vi "Shooter and Reload.vi"(0 "Shooter at bottom limit":T5, 5 "Winch Shifter Servo":T1={"DeviceStatus"={"status"=FALSE, "code"=0, "source"=""}, "Digital Module"=enum."Digital Module 1", "PWM Channel"=enum."Invalid", "DeadBand"={"Name"="", "maxPositivePwm"=0, "minPositivePwm"=0, "centerPwm"=0, "maxNegativePwm"=0, "minNegativePwm"=0, "angularRange"=0}}, 7 "LatchControlDevRef":T8={"DeviceStatus"={"status"=FALSE, "code"=0, "source"=""}, "Type"=enum."PWM", "PWM"={"Digital Module"=enum."Digital Module 1", "PWM Channel"=enum."Invalid", "DeadBand"={"Name"="", "maxPositivePwm"=0, "minPositivePwm"=0, "centerPwm"=0, "maxNegativePwm"=0, "minNegativePwm"=0, "angularRange"=0}}, "CAN"={"Device Number"=0, "Control Mode"=enum."Percent VBus", "Semaphore"=refnum, "Max Vout"=12.0}, "Invert"=FALSE, "TransformRef"=refnum, "InvTransformRef"=refnum}, 9 "ServoDeviceRef":T1={"DeviceStatus"={"status"=FALSE, "code"=0, "source"=""}, "Digital Module"=enum."Digital Module 1", "PWM Channel"=enum."Invalid", "DeadBand"={"Name"="", "maxPositivePwm"=0, "minPositivePwm"=0, "centerPwm"=0, "maxNegativePwm"=0, "minNegativePwm"=0, "angularRange"=0}}, 11 "ShooterWinchRef":T8={"DeviceStatus"={"status"=FALSE, "code"=0, "source"=""}, "Type"=enum."PWM", "PWM"={"Digital Module"=enum."Digital Module 1", "PWM Channel"=enum."Invalid", "DeadBand"={"Name"="", "maxPositivePwm"=0, "minPositivePwm"=0, "centerPwm"=0, "maxNegativePwm"=0, "minNegativePwm"=0, "angularRange"=0}}, "CAN"={"Device Number"=0, "Control Mode"=enum."Percent VBus", "Semaphore"=refnum, "Max Vout"=12.0}, "Invert"=FALSE, "TransformRef"=refnum, "InvTransformRef"=refnum}, 12 "Shooter Latch Sensors":T7) -> ()   [LabVIEW 2014]
uses:
  <vilib>/Rock Robotics/WPI/DigitalInput/WPI_DigitalInputDevRef.ctl
  <vilib>/Rock Robotics/SystemInterfaces/DIO/FPGA_DIOChannel.ctl
  <vilib>/Rock Robotics/SystemInterfaces/Typedef/FPGA_TypedefDigitalModule.ctl
  <vilib>/Rock Robotics/WPI/MotorControl/WPI_MotorControlDeviceRef.ctl
  <vilib>/Rock Robotics/SystemInterfaces/DIO/FPGA_DIOPWMChannel.ctl
  <vilib>/Rock Robotics/WPI/PWM/WPI_PWMDeadband.ctl
  <vilib>/Rock Robotics/WPI/CAN/Jaguar/SubVIs/WPI_CANJaguar_ControlMode.ctl
  <vilib>/Rock Robotics/WPI/PWM/WPI_PWMTransform_ConPane.ctl
  <vilib>/Rock Robotics/WPI/PWM/Servo/WPI_ServoDeviceRef.ctl
  Shoot and reload typedef.ctl
  Events.vi
panel:
  out "Shooter Latch Sensor Bottom":bool
  out "Shooter Latch Sensor Top":bool
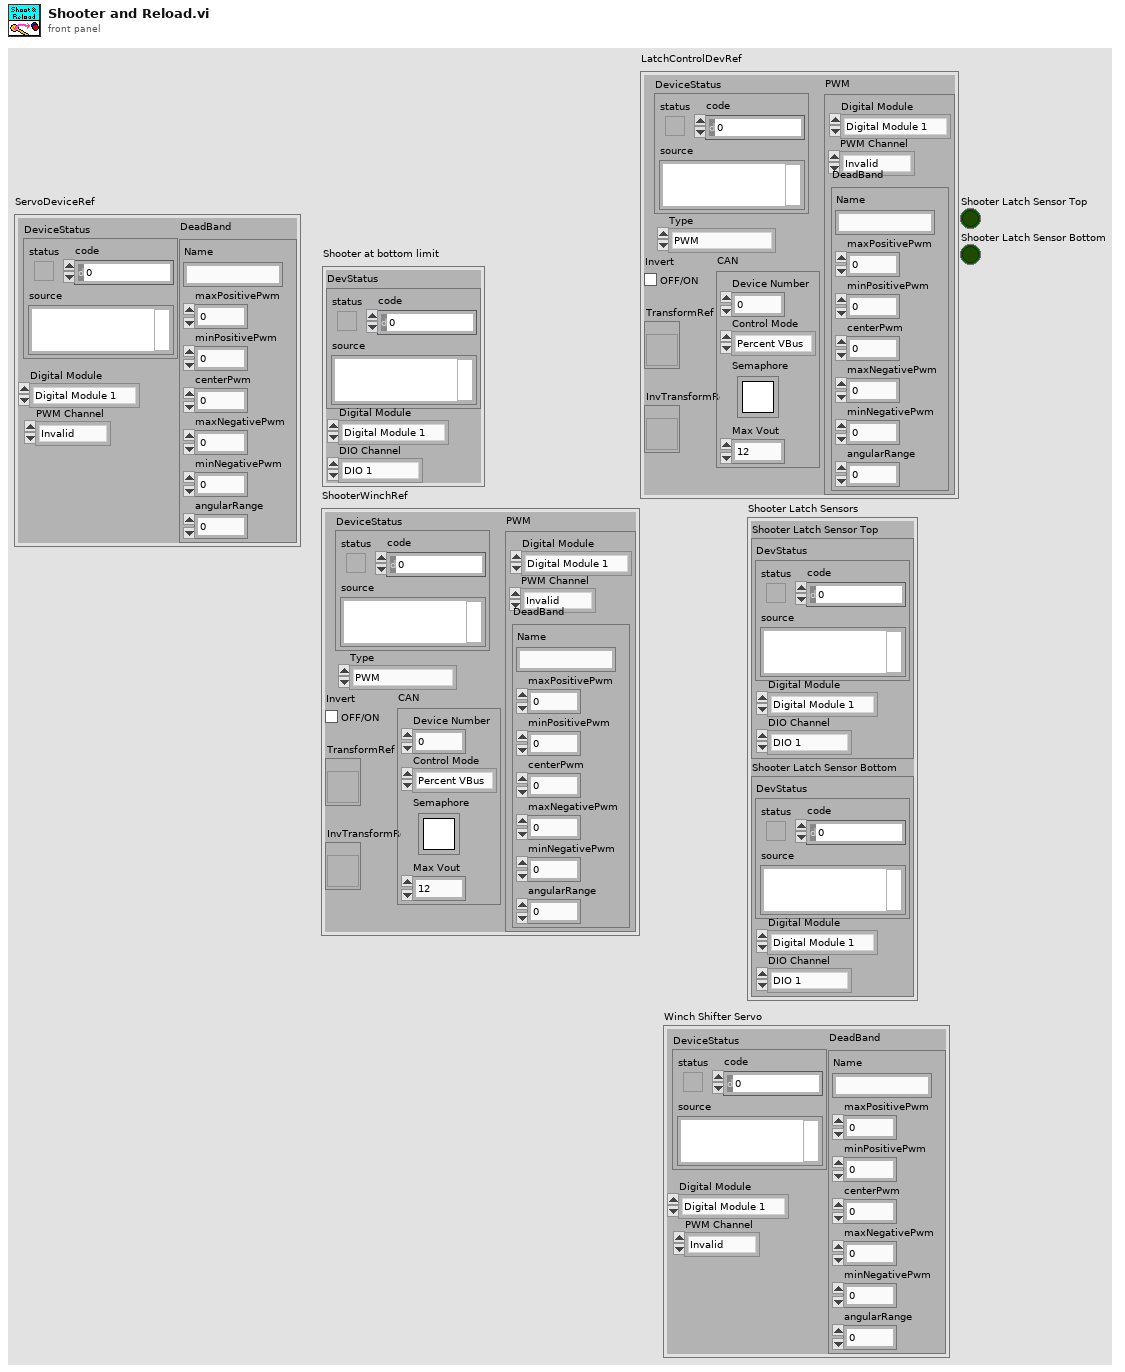
[diagram p1: front panel]
types:
  T1 = typedef "WPI_ServoDeviceRef.ctl" = cluster{"DeviceStatus":errorcluster, "Digital Module":T2, "PWM Channel":T3, "DeadBand":T4}
  T2 = typedef "FPGA_TypedefDigitalModule.ctl" = enum16{"Digital Module 1", "Digital Module 2"}
  T3 = typedef "FPGA_DIOPWMChannel.ctl" = enum8{"PWM 1", "PWM 2", "PWM 3", "PWM 4", "PWM 5", "PWM 6", "PWM 7", "PWM 8", "PWM 9", "PWM 10", "Invalid"}
  T4 = typedef "WPI_PWMDeadband.ctl" = cluster{"Name":string, "maxPositivePwm":i32, "minPositivePwm":i32, "centerPwm":i32, "maxNegativePwm":i32, "minNegativePwm":i32, "angularRange":u16}
  T5 = typedef "WPI_DigitalInputDevRef.ctl" = cluster{"DevStatus":errorcluster, "DIO Channel":T6, "Digital Module":T2}
  T6 = typedef "FPGA_DIOChannel.ctl" = enum8{"DIO 1", "DIO 2", "DIO 3", "DIO 4", "DIO 5", "DIO 6", "DIO 7", "DIO 8", "DIO 9", "DIO 10", "DIO 11", "DIO 12", "DIO 13", "DIO 14", "Invalid"}
  T7 = cluster{"Shooter Latch Sensor Top":T5, "Shooter Latch Sensor Bottom":T5}
  T8 = typedef "WPI_MotorControlDeviceRef.ctl" = cluster{"DeviceStatus":errorcluster, "Type":enum16{"PWM", "CAN"}, "PWM":cluster{"Digital Module":T2, "PWM Channel":T3, "DeadBand":T4}, "CAN":cluster{"Device Number":u8, "Control Mode":T9, "Semaphore":T10, "Max Vout":dbl}, "Invert":bool, "TransformRef":T11, "InvTransformRef":T11}
  T9 = typedef "WPI_CANJaguar_ControlMode.ctl" = enum8{"Percent VBus", "Current", "Speed", "Position", "Voltage"}
  T10 = typedef "Semaphore RefNum" = refnum<k1>
  T11 = typedef "WPI_PWMTransform_ConPane.ctl" = refnum<vi>
  T12 = typedef "Shoot and reload typedef.ctl" = enum16{"Wait for fire button", "First call", "Release Latch", "Wait for reload to be needed", "Engage gearbox", "Run motor", "Engage latch / Stall motor", "Stop motor", "truss shot servos", "Disengage Gearbox"}
  T13 = cluster{"axis 1":dbl, "axis 2":dbl, "axis 3":dbl, "axis 4":dbl, "axis 5":dbl, "Change Power":dbl}
  T14 = cluster{"Reloading?":bool, "Throw":bool, "Ready?":bool, "Truss throw":bool, "Power is high?":bool, "Automatic relaod?":bool, "Manuall servo":bool}
  T15 = typedef "Eventgrab.ctl" = cluster{"Grab":bool, "GroundPass":bool, "Test Aqaure":dbl, "Shoulder up or down?":bool, "Auton drag":bool}
  T16 = cluster{"Shooter latch power":dbl, "Shooter winch power":dbl, "Shooter gearbox servo angles disengaged":i32, "Shooter gearbox servo angles engaged":i32, "Shooter winch power while stalling":dbl, "Exponential Drive Exponent":dbl}
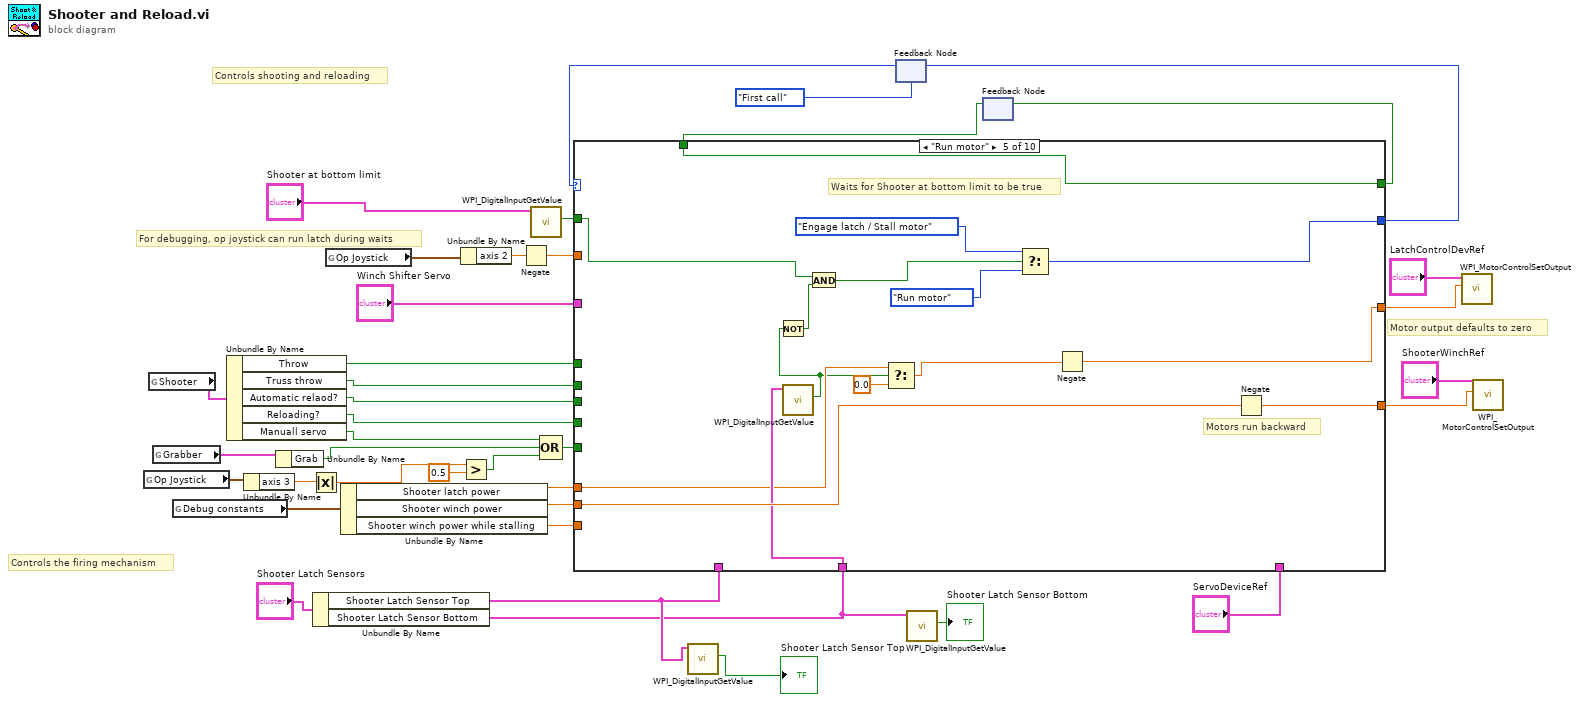
[diagram p0: block diagram]
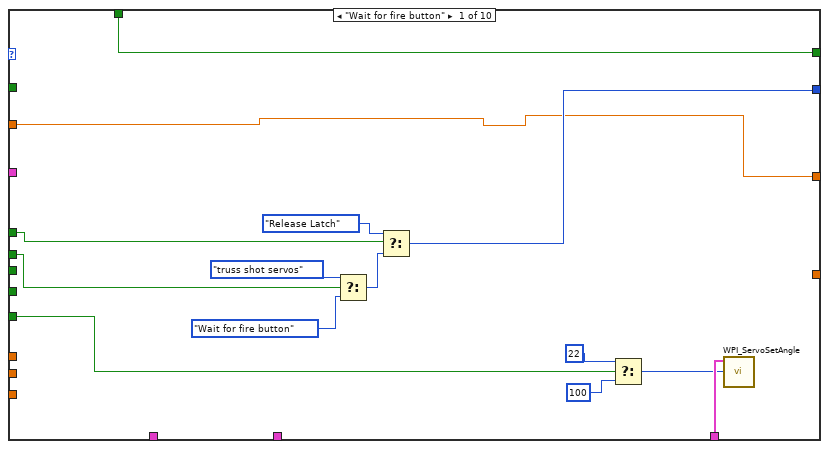
[diagram p2: hidden frame]
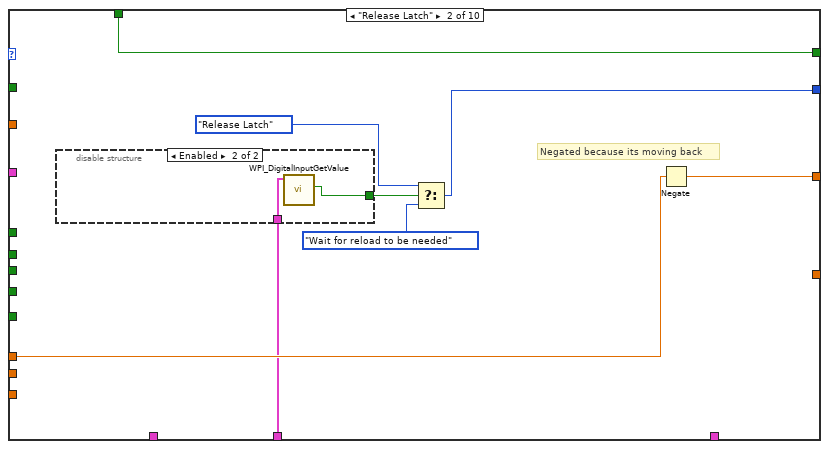
[diagram p3: hidden frame]
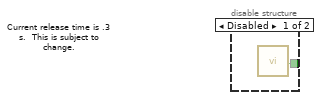
[diagram p4: hidden frame]
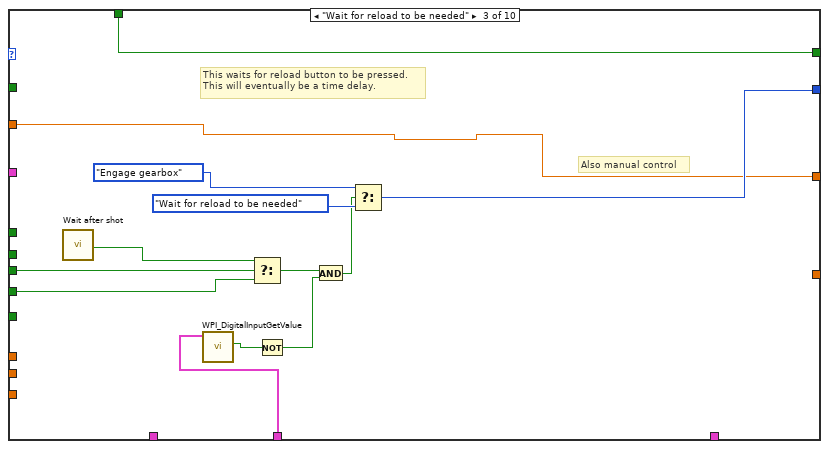
[diagram p5: hidden frame]
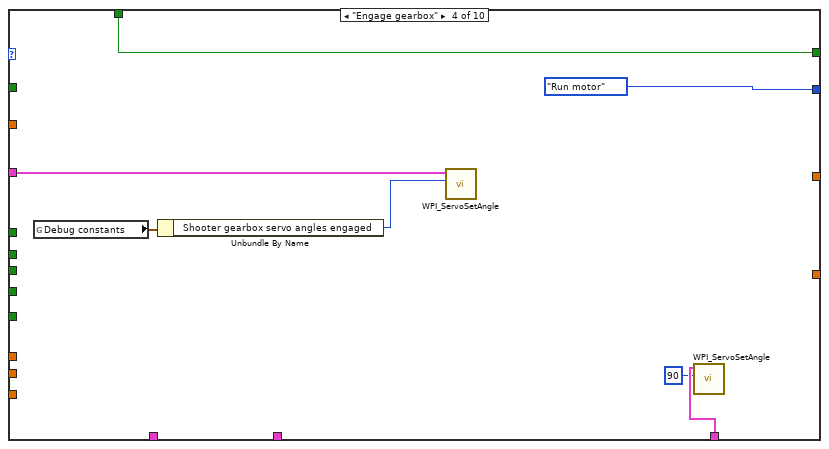
[diagram p6: hidden frame]
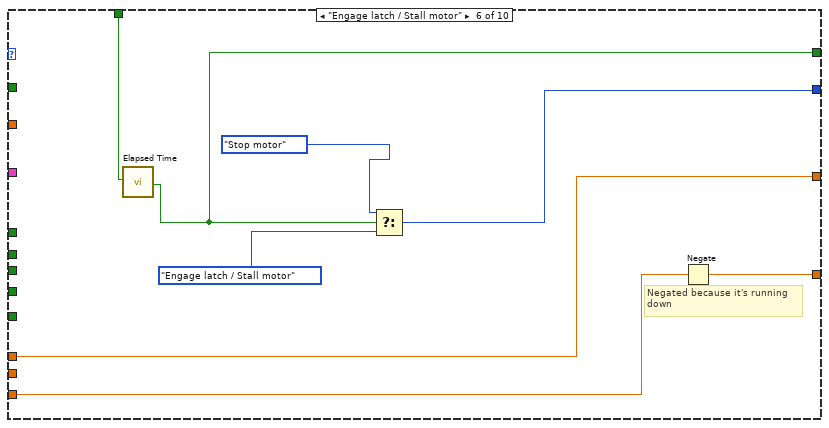
[diagram p7: hidden frame]
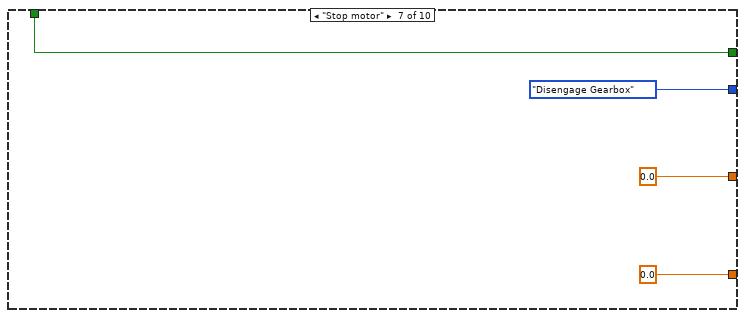
[diagram p8: hidden frame]
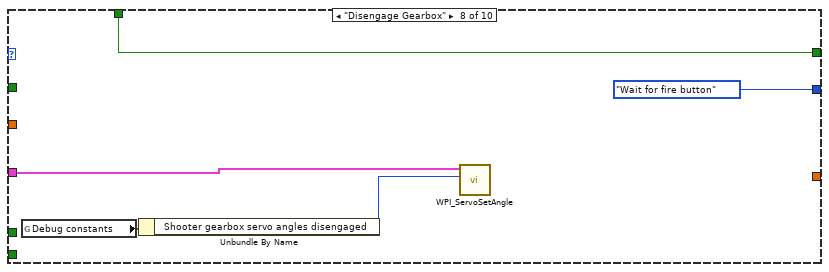
[diagram p9: hidden frame]
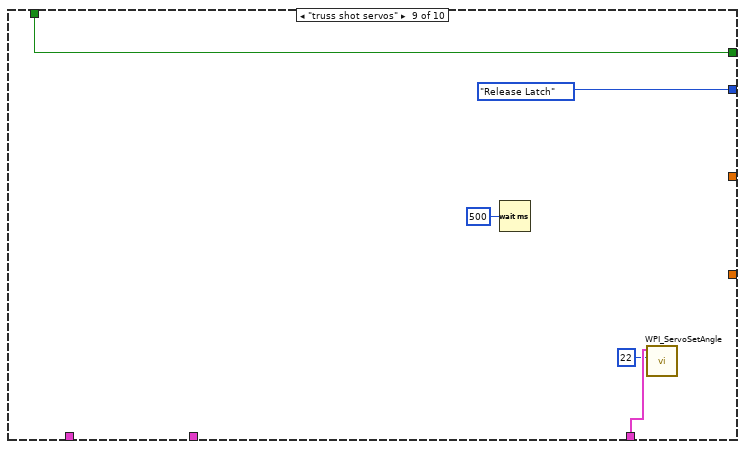
[diagram p10: hidden frame]
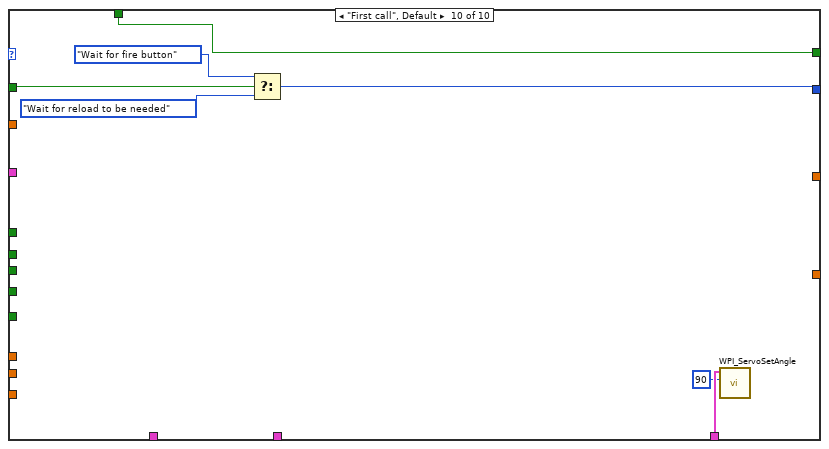
[diagram p11: hidden frame]
diagram:
  # "For debugging, op joystick can run latch during waits"
  # "Motor output defaults to zero"
  # "Controls the firing mechanism"
  # "Controls shooting and reloading"
  n1 = global read "Events.vi" "Op Joystick"() -> (w10:T13)
  n2 = global read "Events.vi" "Shooter"() -> (w39:T14)
  n3 = global read "Events.vi" "Grabber"() -> (w11:T15)
  n4 = global read "Events.vi" "Debug constants"() -> (w24:T16)
  n5 = Unbundle By Name(w39) -> ("Throw"=w14:bool, "Truss throw"=w13:bool, "Automatic relaod?"=w17:bool, "Reloading?"=w25:bool, "Manuall servo"=w6:bool)
  n6 = Unbundle By Name(w10) -> ("axis 3"=w9:dbl)
  n7 = Unbundle By Name(w11) -> ("Grab"=w5:bool)
  n8 = Absolute Value(x=w9) -> (abs(x)=w8:dbl)
  n9 = Unbundle By Name("Shooter Latch Sensors") -> ("Shooter Latch Sensor Top"=w18:T5, "Shooter Latch Sensor Bottom"=w16:T5)
  n10 = global read "Events.vi" "Op Joystick"() -> (w28:T13)
  n11 = Unbundle By Name(w24) -> ("Shooter latch power"=w23:dbl, "Shooter winch power"=w22:dbl, "Shooter winch power while stalling"=w21:dbl)
  n12 = Unbundle By Name ("ubn")(w28) -> ("axis 2"=w27:dbl)
  n13 = Greater?(x=w8, y=0.5) -> (0:w4:bool)
  n14 = Negate(x=w27) -> (-x=w26:dbl)
  n15 = call <vilib>:"WPI_DigitalInputGetValue.vi"("DigitalInputDevRef"="Shooter at bottom limit") -> ("Value"=w36:bool)  [unwired: 8 in, 2 out]
  n16 = Compound Arithmetic op=OR(w6, w5, w4) -> (w3:bool)
  n17 = call <vilib>:"WPI_DigitalInputGetValue.vi"("DigitalInputDevRef"=w18) -> ("Value"=→"Shooter Latch Sensor Top":bool)  [unwired: 8 in, 2 out]
  n18 = feedback #1(Shoot_and_reload_typedef."First call") -> (w34:T12)
  n19 = call <vilib>:"WPI_DigitalInputGetValue.vi"("DigitalInputDevRef"=w16) -> ("Value"=→"Shooter Latch Sensor Bottom":bool)  [unwired: 8 in, 2 out]
  n20 = feedback #2() -> (w2:bool)  [unwired: 1 in]
  n21 = case shown="\"Run motor\"" w34 {
    tunnel: w36 -> [_ _ _ _ w93 _ _ _ _ w128]
    tunnel: [w53 w60 w77 Shoot_and_reload_typedef."Run motor" w99 w107 Shoot_and_reload_typedef."Disengage Gearbox" ("f") Shoot_and_reload_typedef."Wait for fire button" ("f") Shoot_and_reload_typedef."Release Latch" ("f") w127] -> w35
    tunnel: [w41 w55 w66 _ w86 w104 0.0 _ _ _] -> w32
    tunnel: w25 -> [_ _ w74 _ _ _ _ _ _ _]
    tunnel: "Winch Shifter Servo" -> [_ _ _ w84 _ _ _ w116 _ _]
    tunnel: [_ _ _ _ w95 w106 0.0 ("Output") _ _ _] -> w29
    tunnel: w26 -> [w41 _ w66 _ _ _ _ _ _ _]
    tunnel: w23 -> [_ w57 _ _ w91 w104 _ _ _ _]
    tunnel: w22 -> [_ _ _ _ w96 _ _ _ _ _]
    tunnel: w21 -> [_ _ _ _ _ w105 _ _ _ _]
    tunnel: w18 -> [_ _ _ _ _ _ _ _ _ _]
    tunnel: w16 -> [_ w56 w67 _ w94 _ _ _ _ _]
    tunnel: w17 -> [_ _ w73 _ _ _ _ _ _ _]
    tunnel: w14 -> [w51 _ _ _ _ _ _ _ _ _]
    tunnel: w13 -> [w47 _ _ _ _ _ _ _ _ _]
    tunnel: "ServoDeviceRef" -> [w46 _ _ w80 _ _ _ _ w121 w124]
    tunnel: w3 -> [w42 _ _ _ _ _ _ _ _ _]
    tunnel: [w40 w54 w65 w78 w85 w101 w108 w112 w117 w122] -> w1
    tunnel: w2 -> [w40 w54 w65 w78 w85 w100 w108 w112 w117 w122]
    frame "Wait for fire button" {
      n22 = Select(t=Shoot_and_reload_typedef."truss shot servos", s=w47, f=Shoot_and_reload_typedef."Wait for fire button") -> (s? t:f=w49:T12)
      n23 = Select(t=Shoot_and_reload_typedef."Release Latch", s=w51, f=w49) -> (s? t:f=w53:T12)
      n24 = Select(t=22, s=w42, f=100) -> (s? t:f=w44:i32)
      n25 = call <vilib>:"WPI_ServoSetAngle.vi"("Angle"=w44, "ServoDeviceRef"=w46) -> ()  [unwired: 8 in, 2 out]
    }
    frame "Release Latch" {
      # "Negated because its moving back"
      n26 = disable-structure shown="Enabled" {
        disable-tunnel: [w62 w64] -> w61
        disable-tunnel: w56 -> [_ w63]
        frame Disabled {
          n27 = call "Current release time is .3 s.  This is subject to change."() -> ("Time has Elapsed"=w62:bool)  [unwired: 12 in, 7 out]
        }
        frame Enabled {
          n28 = call <vilib>:"WPI_DigitalInputGetValue.vi"("DigitalInputDevRef"=w63) -> ("Value"=w64:bool)  [unwired: 8 in, 2 out]
        }
      }
      n29 = Select(t=Shoot_and_reload_typedef."Release Latch", s=w61, f=Shoot_and_reload_typedef."Wait for reload to be needed") -> (s? t:f=w60:T12)
      n30 = Negate(x=w57) -> (-x=w55:dbl)
    }
    frame "Wait for reload to be needed" {
      # "Also manual control"
      # "This waits for reload button to be pressed.\nThis will eventually be a time delay."
      n31 = call "Wait after shot"() -> ("Time has Elapsed"=w72:bool)  [unwired: 12 in, 7 out]
      n32 = call <vilib>:"WPI_DigitalInputGetValue.vi"("DigitalInputDevRef"=w67) -> ("Value"=w68:bool)  [unwired: 8 in, 2 out]
      n33 = Select(t=w72, s=w73, f=w74) -> (s? t:f=w70:bool)
      n34 = Not(x=w68) -> (.not. x?=w71:bool)
      n35 = And(x=w70, y=w71) -> (x .and. y?=w69:bool)
      n36 = Select(t=Shoot_and_reload_typedef."Engage gearbox", s=w69, f=Shoot_and_reload_typedef."Wait for reload to be needed") -> (s? t:f=w77:T12)
    }
    frame "Engage gearbox" {
      n37 = global read "Events.vi" "Debug constants"() -> (w82:T16)
      n38 = Unbundle By Name(w82) -> ("Shooter gearbox servo angles engaged"=w81:i32)
      n39 = call <vilib>:"WPI_ServoSetAngle.vi"("Angle"=w81, "ServoDeviceRef"=w84) -> ()  [unwired: 8 in, 2 out]
      n40 = call <vilib>:"WPI_ServoSetAngle.vi"("Angle"=90, "ServoDeviceRef"=w80) -> ()  [unwired: 8 in, 2 out]
    }
    frame "Run motor" {
      # "Motors run backward"
      # "Waits for Shooter at bottom limit to be true"
      n41 = call <vilib>:"WPI_DigitalInputGetValue.vi"("DigitalInputDevRef"=w94) -> ("Value"=w89:bool)  [unwired: 8 in, 2 out]
      n42 = Not(x=w89) -> (.not. x?=w88:bool)
      n43 = And(x=w93, y=w88) -> (x .and. y?=w92:bool)
      n44 = Select(t=w91, s=w89, f=0.0) -> (s? t:f=w87:dbl)
      n45 = Select(t=Shoot_and_reload_typedef."Engage latch / Stall motor", s=w92, f=Shoot_and_reload_typedef."Run motor") -> (s? t:f=w99:T12)
      n46 = Negate(x=w87) -> (-x=w86:dbl)
      n47 = Negate(x=w96) -> (-x=w95:dbl)
    }
    frame "Engage latch / Stall motor" {
      # "Negated because it's running\ndown"
      n48 = call "Elapsed Time"("Reset"=w100) -> ("Time has Elapsed"=w101:bool)  [unwired: 11 in, 7 out]
      n49 = Select(t=Shoot_and_reload_typedef."Stop motor", s=w101, f=Shoot_and_reload_typedef."Engage latch / Stall motor") -> (s? t:f=w107:T12)
      n50 = Negate(x=w105) -> (-x=w106:dbl)
    }
    frame "Stop motor" {
    }
    frame "Disengage Gearbox" {
      n51 = global read "Events.vi" "Debug constants"() -> (w114:T16)
      n52 = Unbundle By Name(w114) -> ("Shooter gearbox servo angles disengaged"=w113:i32)
      n53 = call <vilib>:"WPI_ServoSetAngle.vi"("Angle"=w113, "ServoDeviceRef"=w116) -> ()  [unwired: 8 in, 2 out]
    }
    frame "truss shot servos" {
      n54 = Wait (ms)(milliseconds to wait=u32 500) -> ()  [unwired: 1 out]
      n55 = call <vilib>:"WPI_ServoSetAngle.vi"("Angle"=22, "ServoDeviceRef"=w121) -> ()  [unwired: 8 in, 2 out]
    }
    frame "First call", Default {
      n56 = Select(t=Shoot_and_reload_typedef."Wait for fire button", s=w128, f=Shoot_and_reload_typedef."Wait for reload to be needed") -> (s? t:f=w127:T12)
      n57 = call <vilib>:"WPI_ServoSetAngle.vi"("Angle"=90, "ServoDeviceRef"=w124) -> ()  [unwired: 8 in, 2 out]
    }
  }
  n58 = feedback-in #1(w35) -> ()
  n59 = feedback-in #2(w1) -> ()
  n60 = call <vilib>:"WPI_MotorControlSetOutput.vi"("Output"=w32, "MotorControlDevRef"="LatchControlDevRef") -> ()  [unwired: 7 in, 3 out]
  n61 = call <vilib>:"WPI_MotorControlSetOutput.vi"("Output"=w29, "MotorControlDevRef"="ShooterWinchRef") -> ()  [unwired: 7 in, 3 out]
